vi "ToREALCluster.vi"(0 "Element Names (destination) out":string[](array[string]), 1 "variant  (source)":variant, 2 "Array":string[](array[string]), 3 "error out":errorcluster, 4 "variant (destination)":variant) -> (5 "variant (destination) out":variant, 6 "error out 2":errorcluster)   [LabVIEW 2011]
uses:
  OnOffTypeDef.ctl
panel:
  out "dt":u32
  out "Numeric":i32
  out "Array 2":bool[](array[boolean])
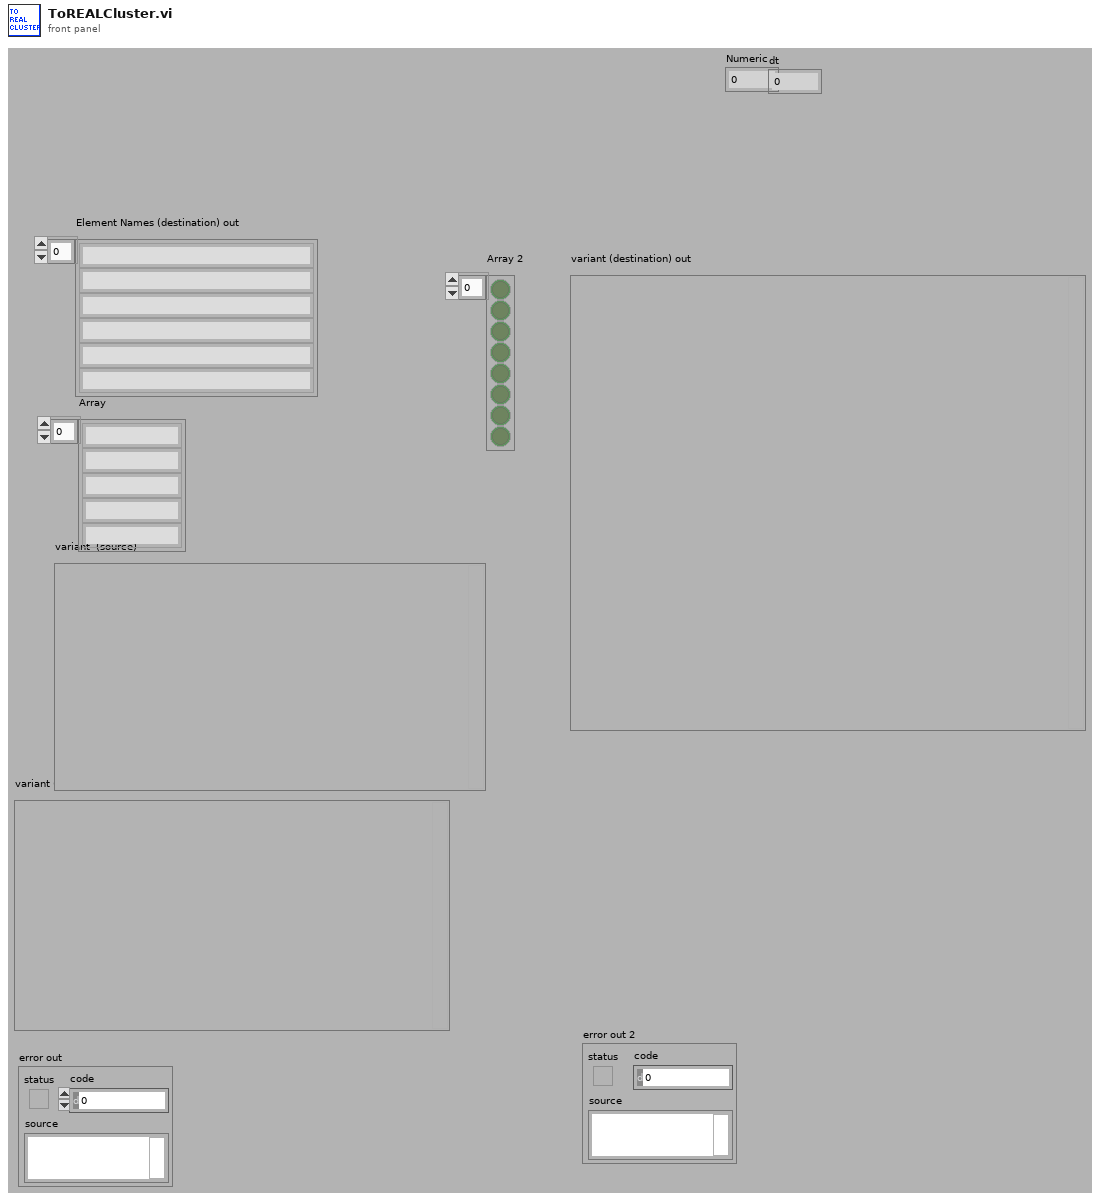
[diagram p1: front panel]
types:
  T1 = typedef "OnOffTypeDef.ctl" = enum16{"off", "on"}
  T2 = typedef "Type Descriptor Enumeration__ogtk.ctl" = enum8{"<Null>", "I8", "I16", "I32", "I64", "U8", "U16", "U32", "U64", "SGL", "DBL", "EXT", "CSG", "CDB", "CXT", "0x0F", "0x10", "0x11", "0x12", "0x13", "0x14", "Enum U8", "Enum U16", "Enum U32", "Enum U64", "SGL PQ", "DBL PQ", "EXT PQ", "CSG PQ", "CDB PQ", "CXT PQ", "0x1F", "0x20", "Boolean", "0x22", "0x23", "0x24", "0x25", "0x26", "0x27", "0x28", "0x29", "0x2A", "0x2B", "0x2C", "0x2D", "0x2E", "0x2F", "String", "0x31", "Path", "Pict", "0x34", "0x35", "0x36", "DAQ", "0x38", "0x39", "0x3A", "0x3B", "0x3C", "0x3D", "0x3E", "0x3F", "Array", "0x41", "0x42", "0x43", "0x44", "0x45", "0x46", "0x47", "0x48", "0x49", "0x4A", "0x4B", "0x4C", "0x4D", "0x4E", "0x4F", "Cluster", "0x51", "0x52", "Variant", "Waveform", "0x55", "0x56", "0x57", "0x58", "0x59", "0x5A", "0x5B", "0x5C", "0x5D", "0x5E", "0x5F", "0x60", "0x61", "0x62", "0x63", "0x64", "0x65", "0x66", "0x67", "0x68", "0x69", "0x6A", "0x6B", "0x6C", "0x6D", "0x6E", "0x6F", "Refnum"}
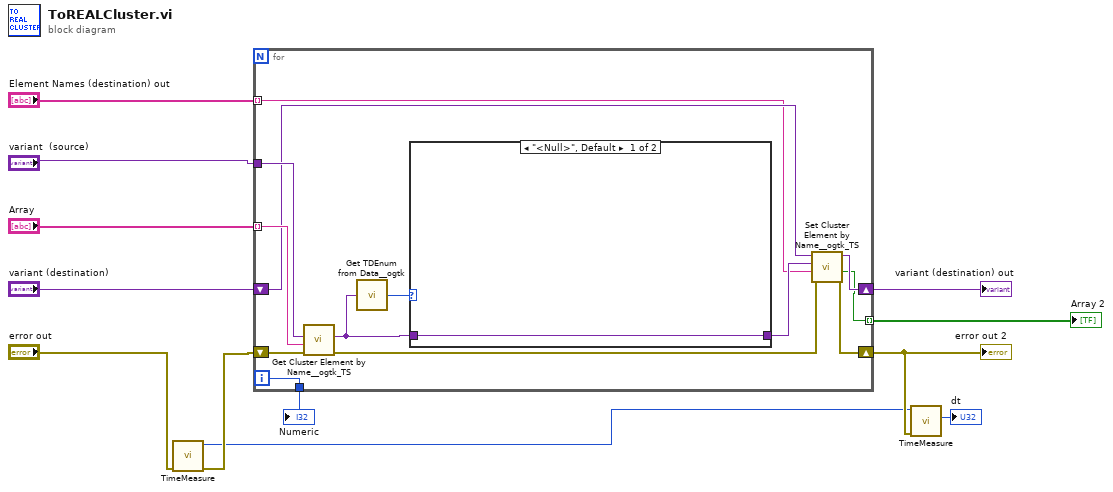
[diagram p0: block diagram]
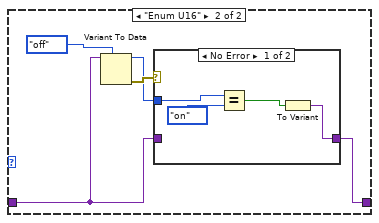
[diagram p2: hidden frame]
diagram:
  n1 = call "TimeMeasure.vi"("error in (no error)"="error out") -> ("error out"=w4:errorcluster, "time out"=w2:u32)  [unwired: 8 in, 1 out]
  n2 = for {
    tunnel: "Array" -> [w25] mode=indexing
    tunnel: "variant  (source)" -> [w24]
    shift-right: [w17] -> w8
    shift-left: "variant (destination)" -> [w20]
    shift-right: [w15] -> w3
    shift-left: w4 -> [w21]
    tunnel: "Element Names (destination) out" -> [w18] mode=indexing
    tunnel: [w14] -> w9 mode=indexing
    tunnel: [w13] -> w6
    i -> [w13]
    n3 = call "Get Cluster Element by Name__ogtk_TS.vi"("error in (no error)"=w21, "Element Name"=w25, "Cluster"=w24) -> ("error out"=w16:errorcluster, "VElement"=w23:variant)  [unwired: 6 in, 1 out]
    n4 = call "Get TDEnum from Data__ogtk.vi"("Data"=w23) -> ("Type Descriptor Enumeration"=w22:T2)  [unwired: 4 in]
    n5 = case shown="\"<Null>\", Default" w22 {
      tunnel: [w26 w29] -> w19
      tunnel: w23 -> [w26 w28]
      frame "<Null>", Default {
      }
      frame "Enum U16" {
        n6 = Variant To Data(type=OnOffTypeDef."off" ("Save"), Variant=w28) -> (data=w30:T1, error out=w31:errorcluster)  [unwired: 1 in]
        n7 = case shown="No Error" w31 {
          tunnel: w30 -> [w34 _]
          tunnel: [w35 w36] -> w29
          tunnel: w28 -> [_ w36]
          frame No Error {
            n8 = Equal?(x=w34, y=OnOffTypeDef."on" ("Save")) -> (x = y?=w32:bool)
            n9 = To Variant(anything=w32) -> (Variant=w35:variant)
          }
          frame Error {
          }
        }
      }
    }
    n10 = call "Set Cluster Element by Name__ogtk_TS.vi"("error in (no error)"=w16, "Element Name (\"\": New Element Data Name)"=w18, "New Element Value"=w19, "Cluster"=w20) -> ("error out"=w15:errorcluster, "found?"=w14:bool, "VCluster out"=w17:variant)  [unwired: 5 in]
  }
  "error out 2" <- w3
  "variant (destination) out" <- w8
  "Array 2" <- w9
  "Numeric" <- w6
  n11 = call "TimeMeasure.vi"("error in (no error)"=w3, "time in"=w2) -> ("dt"=→"dt":u32)  [unwired: 7 in, 2 out]
